vi "Enable Page.vi"(8 "error in (no error)":errorcluster, 10 "Page Index":i32, 11 "Steps in":refnum<class "Steps.lvclass">) -> (0 "error out":errorcluster, 3 "Steps out":refnum<class "Steps.lvclass">)   [LabVIEW 2015, in "Steps.lvclass"]
doc: "<b> </b> <b> </b>\n©2016 Q Software Innovations, LLC (QSI)\nwritten by Quentin Alldredge\nproduced in LabVIEW 2015\n\nsupport@qsoftwareinnovations.com\nwww.qsoftwareinnovations.com\n\nAll rights reserved.\n\nRedistribution and use in source and binary forms, with or without modification, are permitted provided that the following conditions are met:\n\n * Redistributions of source code must retain the above copyright notice, this list of conditions and the following disclaimer.\n * Redistributions in binary form must reproduce the above copyright notice, this list of conditions and the following disclaimer in the documentation and/or other materials provided with the distribution.\n * Neither the name of Q Software Innovations, LLC. nor the names of its contributors may be used to endorse or promote products derived from this software without specific prior written permission.\n\nTHIS SOFTWARE IS PROVIDED BY THE COPYRIGHT HOLDERS AND CONTRIBUTORS \"AS IS\" AND ANY EXPRESS OR IMPLIED WARRANTIES, INCLUDING, BUT NOT LIMITED TO, THE IMPLIED WARRANTIES OF MERCHANTABILITY AND FITNESS FOR A PARTICULAR PURPOSE ARE DISCLAIMED. IN NO EVENT SHALL THE COPYRIGHT OWNER OR CONTRIBUTORS BE LIABLE FOR ANY DIRECT, INDIRECT, INCIDENTAL, SPECIAL, EXEMPLARY, OR CONSEQUENTIAL DAMAGES (INCLUDING, BUT NOT LIMITED TO, PROCUREMENT OF SUBSTITUTE GOODS OR SERVICES; LOSS OF USE, DATA, OR PROFITS; OR BUSINESS INTERRUPTION) HOWEVER CAUSED AND ON ANY THEORY OF LIABILITY, WHETHER IN CONTRACT, STRICT LIABILITY, OR TORT (INCLUDING NEGLIGENCE OR OTHERWISE) ARISING IN ANY WAY OUT OF THE USE OF THIS SOFTWARE, EVEN IF ADVISED OF THE POSSIBILITY OF SUCH DAMAGE."
uses:
  Steps.lvclass
  Steps.lvclass/Steps.ctl
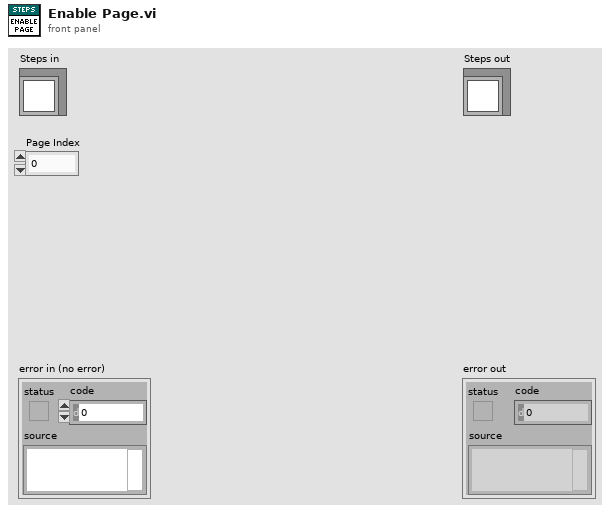
[diagram p1: front panel]
types:
  T1 = enum32{"Page Enabled", "Page Disabled", "Page Disabled & Grayed"}
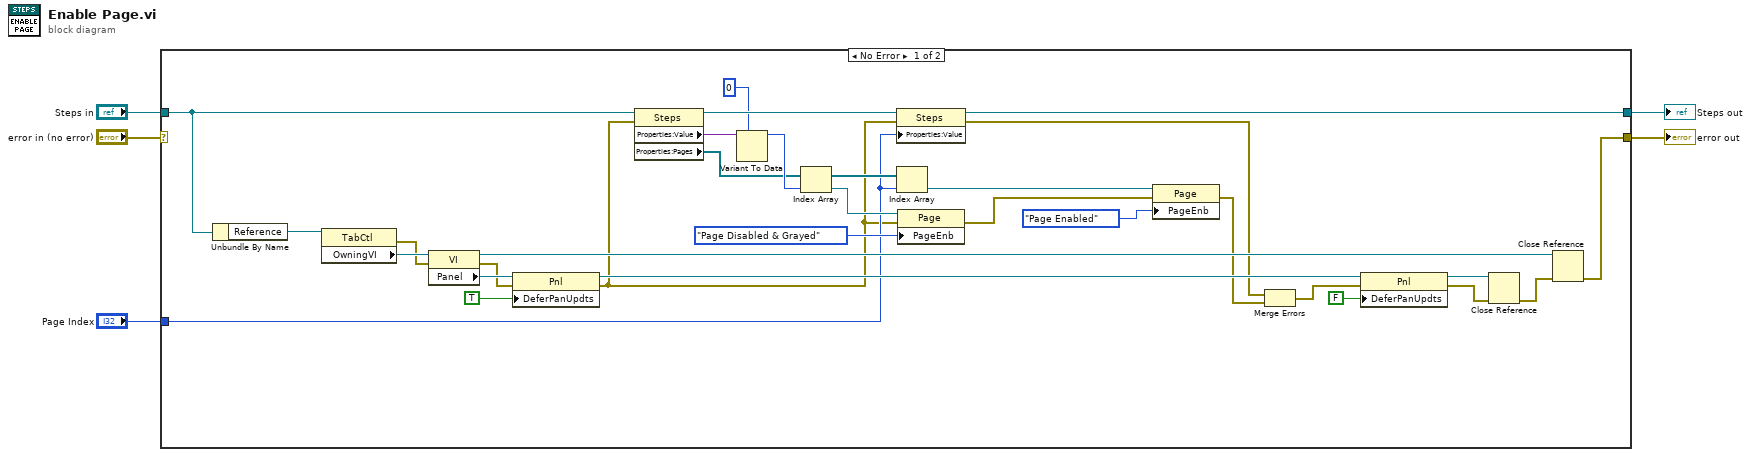
[diagram p0: block diagram]
diagram:
  n1 = case shown="No Error" "error in (no error)" {
    selector: "error in (no error)" -> [_ w37]
    tunnel: [w23 w37] -> w4
    tunnel: [w22 w36] -> w2
    tunnel: "Steps in" -> [w7 w36]
    tunnel: "Page Index" -> [w13 _]
    frame No Error {
      n2 = Unbundle By Name(w7) -> ("Reference"=w6:refnum<vi>)
      n3 = property class="TabCtl"(reference=w6) -> (error out=w33:errorcluster, "OwningVI"=w34:refnum<vi>)  [unwired: 1 in, 1 out]
      n4 = property class="VI"(reference=w34, error in=w33) -> (reference out=w25:refnum<vi>, error out=w31:errorcluster, "Panel"=w32:refnum<vi>)
      n5 = property class="Pnl"(reference=w32, error in=w31, "DeferPanUpdts"=TRUE ("Defer Panel Updates")) -> (reference out=w29:refnum<vi>, error out=w8:errorcluster)
      n6 = property class="Steps"(reference=w7, error in=w8) -> (reference out=w35:refnum<class "Steps.lvclass">, "Properties:Value"=w18:variant, "Properties:Pages"=w14:refnum<vi>[])  [unwired: 1 out]
      n7 = Variant To Data(type=0, Variant=w18) -> (data=w17:i32)  [unwired: 1 in, 1 out]
      n8 = Index Array(array=w14, index=w17) -> (element=w16:refnum<vi>)
      n9 = property class="Steps"(reference=w35, error in=w8, "Properties:Value"=w13) -> (reference out=w22:refnum<class "Steps.lvclass">, error out=w21:errorcluster)
      n10 = Index Array(array=w14, index=w13) -> (element=w12:refnum<vi>)
      n11 = property class="Page"(reference=w16, error in=w8, "PageEnb"=T1."Page Disabled & Grayed" ("Page Enabled State")) -> (error out=w11:errorcluster)  [unwired: 1 out]
      n12 = property class="Page"(reference=w12, error in=w11, "PageEnb"=T1."Page Enabled" ("Page Enabled State")) -> (error out=w9:errorcluster)  [unwired: 1 out]
      n13 = Merge Errors(w21, w9) -> (w20:errorcluster)
      n14 = property class="Pnl"(reference=w29, error in=w20, "DeferPanUpdts"=FALSE ("Defer Panel Updates")) -> (reference out=w27:refnum<vi>, error out=w26:errorcluster)
      n15 = Close Reference(reference=w27, error in (no error)=w26) -> (error out=w24:errorcluster)
      n16 = Close Reference(reference=w25, error in (no error)=w24) -> (error out=w23:errorcluster)
    }
    frame Error {
    }
  }
  "error out" <- w4
  "Steps out" <- w2
